vi "Configure Waveform Polarity.vi"(8 "error in (no error)":errorcluster, 10 "Waveform Polarity (0: Normal)":i32(ring) items=["Normal", "Invert"], 11 "VISA resource name":refnum<visa-resource-name>) -> (0 "error out":errorcluster, 3 "VISA resource name out":refnum<visa-resource-name>)   [LabVIEW 2016, in "Agilent 2000 3000 X-Series.lvlib"]
doc: "Configures the polarity of waveform generator.\n\nNote: This VI is only applicable for 1000 X-Series."
uses:
  Agilent 2000 3000 X-Series.lvlib
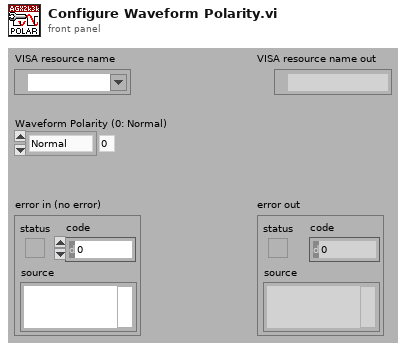
[diagram p1: front panel]
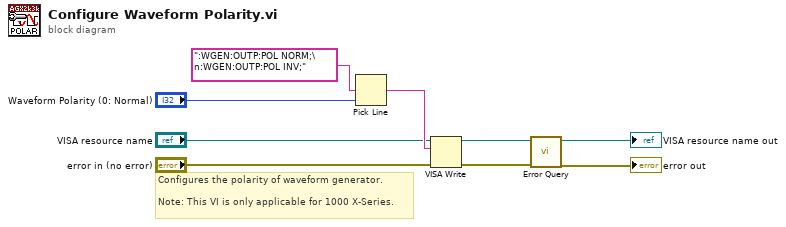
[diagram p0: block diagram]
diagram:
  # "Configures the polarity of waveform generator.\n\nNote: This VI is only applicable for 1000 X-Series."
  n1 = Pick Line(multi-line string=":WGEN:OUTP:POL NORM;\n:WGEN:OUTP:POL INV;", line index="Waveform Polarity (0: Normal)") -> (output string=w7:string)  [unwired: 1 in]
  n2 = VISA Write(VISA resource name="VISA resource name", write buffer=w7, error in (no error)="error in (no error)") -> (VISA resource name out=w4:refnum<visa-resource-name>, error out=w3:errorcluster)  [unwired: 1 out]
  n3 = call "Error Query.vi"("error in (no error)"=w3, "VISA resource name"=w4) -> ("error out"=→"error out":errorcluster, "VISA resource name out"=→"VISA resource name out":refnum<visa-resource-name>)  [unwired: 6 in, 2 out]
